vi "BitChecker.vi"(8 "error in (no error)":errorcluster, 10 "Bit(0-31)":u32, 11 "Input":u32) -> (0 "error out":errorcluster, 2 "IsSet":bool, 3 "Value":i16)   [LabVIEW 2017]
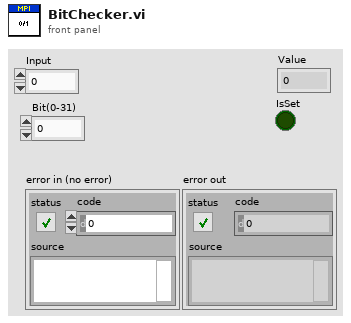
[diagram p1: front panel]
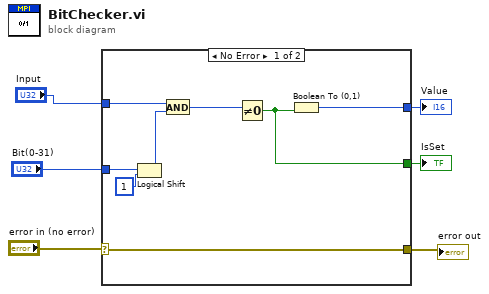
[diagram p0: block diagram]
diagram:
  n1 = case shown="No Error" "error in (no error)" {
    selector: "error in (no error)" -> [w14 w15]
    tunnel: [w14 w15] -> w5
    tunnel: [w12 _] -> w1
    tunnel: [w11 _] -> w2
    tunnel: "Input" -> [w10 _]
    tunnel: "Bit(0-31)" -> [w9 _]
    frame No Error {
      n2 = Logical Shift(y=w9, x=u32 1) -> (x << y=w7:u32)
      n3 = And(x=w10, y=w7) -> (x .and. y?=w13:u32)
      n4 = Not Equal To 0?(x=w13) -> (x != 0?=w11:bool)
      n5 = Boolean To (0,1)(Boolean=w11) -> (0, 1=w12:i16)
    }
    frame Error {
    }
  }
  "error out" <- w5
  "IsSet" <- w2
  "Value" <- w1
